vi "Destroy.vi"(8 "error in (no error)":errorcluster, 10 "Wait for Stop Timeout ms (0)":i32, 11 "Interface in":refnum<data-value>) -> (0 "error out":errorcluster)   [LabVIEW 2018, in "Actor.lvlib" / "Actor-Interface.lvclass"]
uses:
  Actor-Interface.lvclass
  Actor-Interface.lvclass/Actor-Interface.ctl
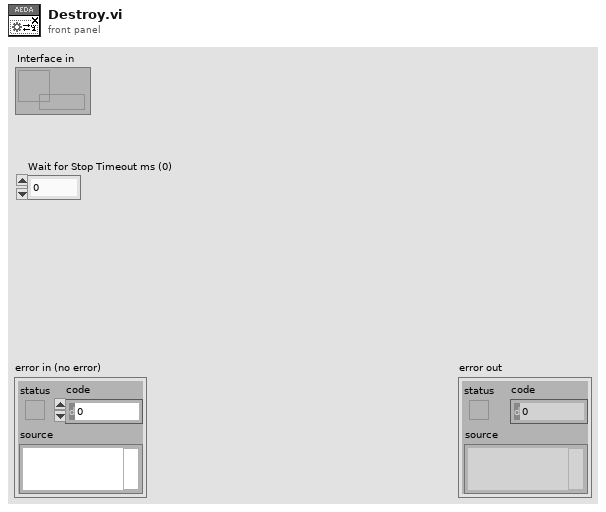
[diagram p1: front panel]
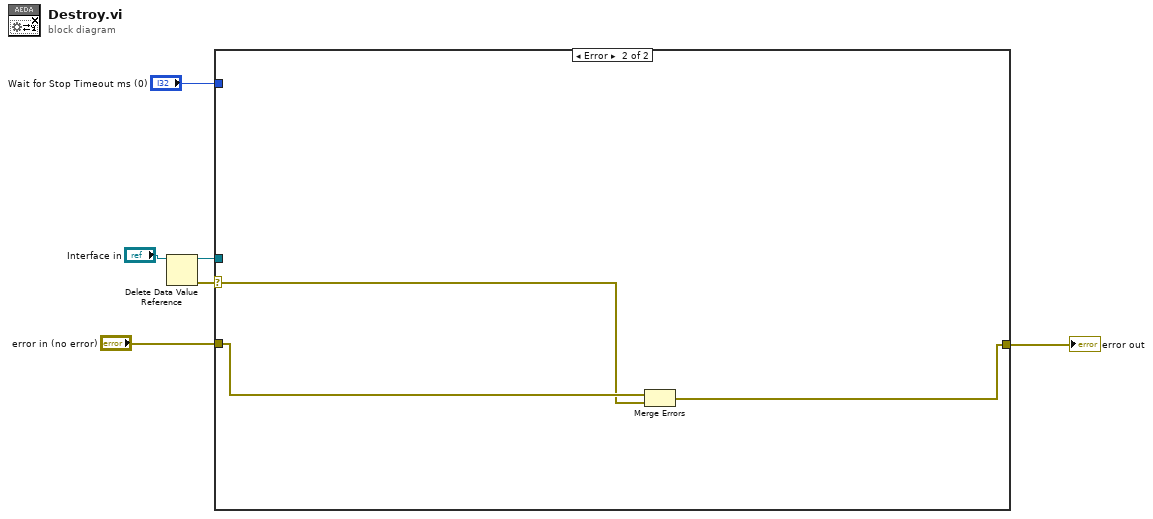
[diagram p0: block diagram]
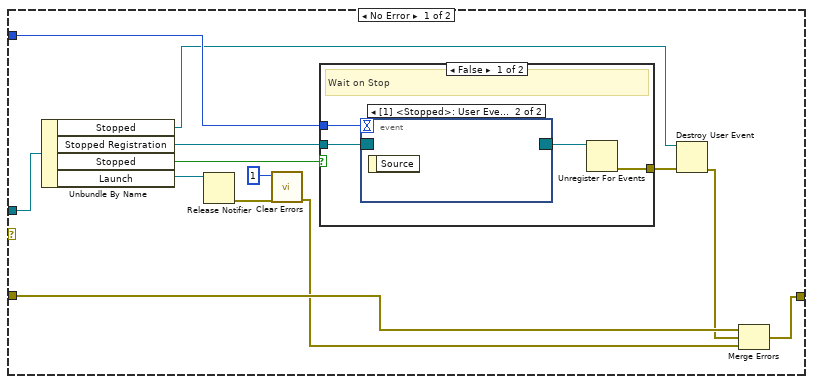
[diagram p2: hidden frame]
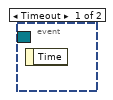
[diagram p3: hidden frame]
diagram:
  n1 = Delete Data Value Reference(data value reference="Interface in") -> (data value=w5:refnum<class "Actor-Interface.lvclass">, error out=w1:errorcluster)  [unwired: 1 in]
  n2 = case shown="Error" w1 {
    selector: w1 -> [_ w25]
    tunnel: w5 -> [w19 _]
    tunnel: "error in (no error)" -> [w18 w26]
    tunnel: "Wait for Stop Timeout ms (0)" -> [w13 _]
    tunnel: [w12 w24] -> w2
    frame No Error {
      n3 = Unbundle By Name(w19) -> ("Stopped"=w8:refnum<user-event>, "Stopped Registration"=w14:refnum<event-registration>, "Stopped"=w15:bool, "Launch"=w11:refnum<notifier>)
      n4 = Release Notifier(notifier=w11) -> (error out=w10:errorcluster)  [unwired: 2 in, 2 out]
      n5 = call <vilib>:"Clear Errors.vi"("error in (no error)"=w10, "specific error code to clear (0: all)"=1) -> ("error out"=w17:errorcluster)  [unwired: 4 in, 1 out]
      n6 = case shown="False" w15 {
        tunnel: w14 -> [w22 _]
        tunnel: w13 -> [w23 _]
        tunnel: [w20 _] -> w9
        frame False {
          # "Wait on Stop"
          n7 = event shown="[1] <Stopped>: User Event" {
            selector: w22 -> [_ _]
            dyn-events: [_ _] -> w21
            timeout: w23 -> [_ _]
            event Timeout {
              n8 = event-data() -> ()  [unwired: 1 in, 1 out]
            }
            event User Event {
              n9 = event-data() -> ()  [unwired: 1 in, 1 out]
            }
          }
          n10 = Unregister For Events(event registration refnum=w21) -> (error out=w20:errorcluster)  [unwired: 1 in]
        }
        frame True {
          # "Already Stopped"
        }
      }
      n11 = Destroy User Event(user event=w8, error in=w9) -> (error out=w7:errorcluster)
      n12 = Merge Errors(w18, w7, w17) -> (w12:errorcluster)
    }
    frame Error {
      n13 = Merge Errors(w26, w25) -> (w24:errorcluster)
    }
  }
  "error out" <- w2
